vi "Semantic_Voice_Array_Msg.vi"(8 "error in (no error)":errorcluster caption="错误输入（无错误）", 10 "值(信号)":T1, 11 "States.lvlib:Guide.lvclass":refnum<class "Guide.lvclass">) -> (0 "error out":errorcluster caption="错误输出", 3 "Process State out":refnum<class "State Actor.lvclass">)   [LabVIEW 2014, in "States.lvlib" / "Guide.lvclass"]
uses:
  Guide.lvclass
  <vilib>/NI/Actors/State Actor/State Actor/State Actor.lvclass
  ctl/Semantic_Voice_Array.ctl
  <vilib>/ActorFramework/Message Enqueuer/Message Enqueuer.lvclass/Message Enqueuer.ctl
  <vilib>/ActorFramework/Message Enqueuer/Enqueue.vi
  <vilib>/ActorFramework/Message Priority Queue/Priority Enqueue.vi
  Global_var/Global_var.vi
  Voice_lib/VoiceControl/Voice.lvclass
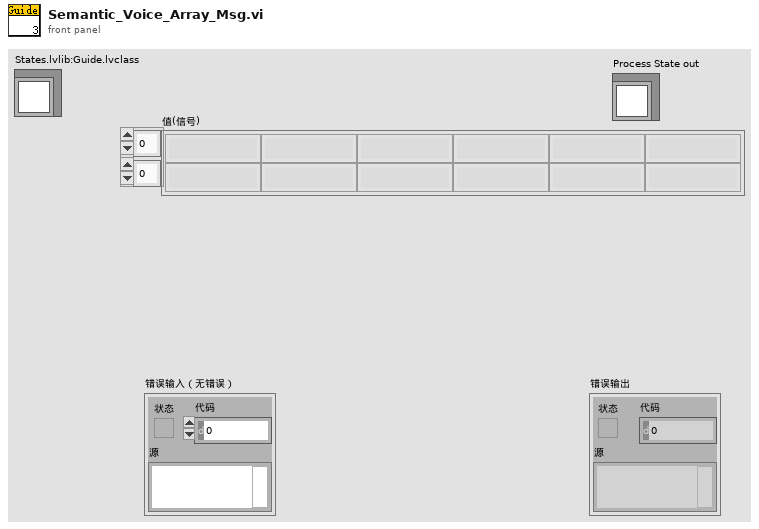
[diagram p1: front panel]
types:
  T1 = typedef "Semantic_Voice_Array.ctl" = string[][]
  T2 = cluster{"起点":string, "终点":string, "动作":string, "方向":string, "距离":string, "速度":string}
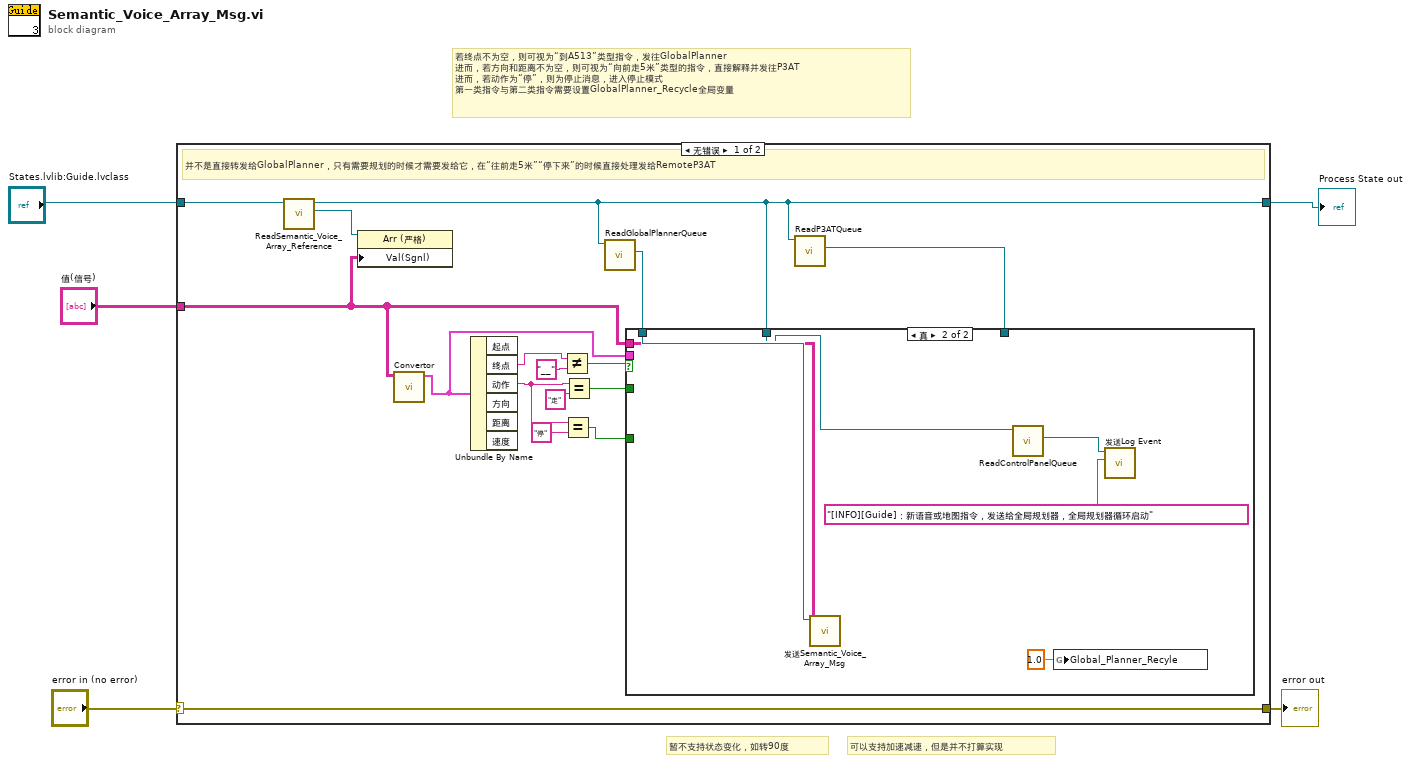
[diagram p0: block diagram]
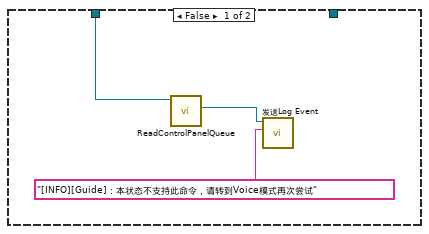
[diagram p2: hidden frame]
diagram:
  # "可以支持加速减速，但是并不打算实现"
  # "暂不支持状态变化，如转90度"
  # "若终点不为空，则可视为“到A513”类型指令，发往GlobalPlanner\n进而，若方向和距离不为空，则可视为“向前走5米”类型的指令，直接解释并发往P3AT\n进而，若动作为“停”，则为停止消息，进入停止模式\n第一类指令与第二类指令需要设置GlobalPlanner_Recycle全局变量"
  n1 = case shown="无错误" "error in (no error)" {
    selector: "error in (no error)" -> [w21 w32]
    tunnel: [w21 w32] -> w4
    tunnel: [w6 w31] -> w3
    tunnel: "States.lvlib:Guide.lvclass" -> [w20 w31]
    tunnel: "值(信号)" -> [w15 _]
    frame No Error {
      # "并不是直接转发给GlobalPlanner，只有需要规划的时候才需要发给它，在“往前走5米”“停下来”的时候直接处理发给RemoteP3AT"
      n2 = call-dynamic "ReadSemantic_Voice_Array_Reference.vi"("CoordinatorState输入"=w20) -> ("Semantic_Voice_Array_Reference"=w19:refnum<vi>, "CoordinatorState输出"=w6:refnum<class "Guide.lvclass">)  [unwired: 8 in, 1 out]
      n3 = property class="Arr (严格)"(reference=w19, "Val(Sgnl)"=w15) -> ()  [unwired: 1 in, 2 out]
      n4 = call "Convertor.vi"("机器人指令数组"=w15) -> ("机器人语音指令数据簇"=w11:T2)  [unwired: 10 in]
      n5 = Unbundle By Name(w11) -> ("终点"=w17:string, "动作"=w9:string)  [unwired: 4 out]
      n6 = Not Equal?(x=w17, y="__") -> (x != y?=w14:bool)
      n7 = Equal?(x=w9, y="停") -> (x = y?=w7:bool)
      n8 = Equal?(x=w9, y="走") -> (x = y?=w12:bool)
      n9 = call-dynamic "ReadGlobalPlannerQueue.vi"("CoordinatorState输入"=w6) -> ("操作者框架:消息待入队列"=w16:refnum<class "Message Enqueuer.lvclass">)  [unwired: 8 in, 2 out]
      n10 = call-dynamic "ReadP3ATQueue.vi"("CoordinatorState输入"=w6) -> ("操作者框架:消息待入队列"=w10:refnum<class "Message Enqueuer.lvclass">)  [unwired: 8 in, 2 out]
      n11 = case shown="真" w14 {
        tunnel: w16 -> [_ w30]
        tunnel: w15 -> [_ w29]
        tunnel: w12 -> [_ _]
        tunnel: w11 -> [_ _]
        tunnel: w10 -> [_ _]
        tunnel: w7 -> [_ _]
        tunnel: w6 -> [w22 w26]
        frame False {
          n12 = call-dynamic "ReadControlPanelQueue.vi"("CoordinatorState输入"=w22) -> ("操作者框架:消息待入队列"=w24:refnum<class "Message Enqueuer.lvclass">)  [unwired: 8 in, 2 out]
          n13 = call "发送Log Event.vi"("Event Text"="[INFO][Guide]：本状态不支持此命令，请转到Voice模式再次尝试", "消息待入队列"=w24) -> ()  [unwired: 8 in, 2 out]
        }
        frame True {
          n14 = call "发送Semantic_Voice_Array_Msg.vi"("值(信号)"=w29, "消息待入队列"=w30) -> ()  [unwired: 8 in, 2 out]
          n15 = call-dynamic "ReadControlPanelQueue.vi"("CoordinatorState输入"=w26) -> ("操作者框架:消息待入队列"=w28:refnum<class "Message Enqueuer.lvclass">)  [unwired: 8 in, 2 out]
          n16 = global write "Global_var.vi" "Global_Planner_Recyle"(1.0 ("Global_Planner_Recyle")) -> ()
          n17 = call "发送Log Event.vi"("Event Text"="[INFO][Guide]：新语音或地图指令，发送给全局规划器，全局规划器循环启动", "消息待入队列"=w28) -> ()  [unwired: 8 in, 2 out]
        }
      }
    }
    frame Error {
    }
  }
  "error out" <- w4
  "Process State out" <- w3
